vi "createBoolean.vi"(8 "error in (no error)":errorcluster, 10 "bool":bool, 11 "IBoolean in":refnum<class "IBoolean.lvclass">) -> (0 "error out":errorcluster, 3 "IBoolean out":refnum<class "IBoolean.lvclass">)   [LabVIEW 2022 SP3, in "openDAQ.lvlib" / "daqCoreTypes.lvlib" / "IBoolean.lvclass"]
uses:
  <instrlib>/openDAQ/Public/Classes/daqCoreTypes/IBoolean/IBoolean.lvclass
  C:/Program Files (x86)/National Instruments/LabVIEW 2022/instr.lib/openDAQ/Public/Classes/IBaseObject/IBaseObject.lvclass
  <instrlib>/openDAQ/Public/Classes/IBaseObject/IBaseObject.lvclass/IBaseObject.ctl
  <instrlib>/openDAQ/Public/Classes/IBaseObject/Accessor/Read reference.vi
  <instrlib>/openDAQ/Public/Classes/IBaseObject/Accessor/Write reference.vi
  <instrlib>/openDAQ/Binaries/Windows/x86/copendaq32.dll
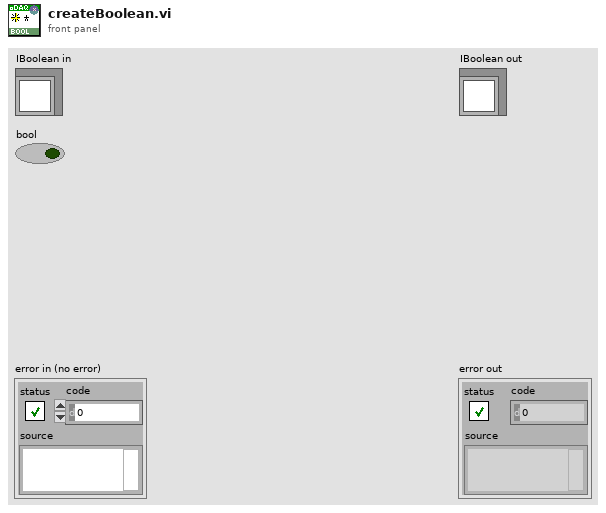
[diagram p1: front panel]
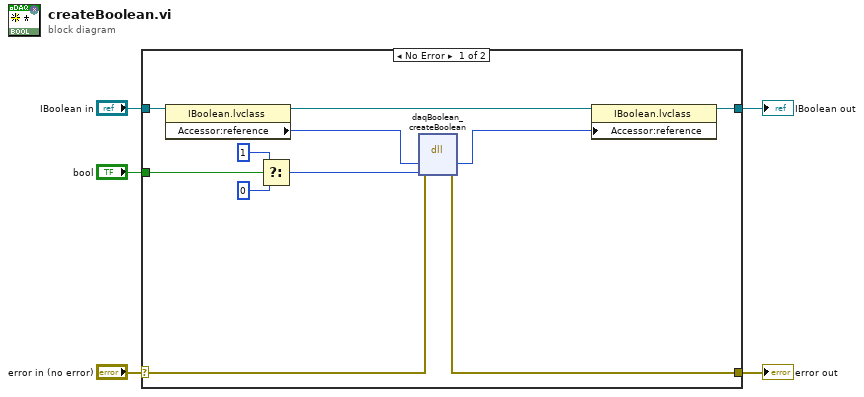
[diagram p0: block diagram]
diagram:
  n1 = case shown="No Error" "error in (no error)" {
    selector: "error in (no error)" -> [w16 w18]
    tunnel: [w15 w18] -> w4
    tunnel: [w13 w17] -> w2
    tunnel: "IBoolean in" -> [w14 w17]
    tunnel: "bool" -> [w9 _]
    frame No Error {
      n2 = property class="IBoolean.lvclass"(reference=w14) -> (reference out=w12:refnum<class "IBoolean.lvclass">, "Accessor:reference"=w11:i64)  [unwired: 1 in, 1 out]
      n3 = Select(t=i64 1 ("value"), s=w9, f=i64 0 ("value")) -> (s? t:f=w6:i64)
      n4 = dll-call lib="C:/Program Files (x86)/National Instruments/LabVIEW 2022/instr.lib/openDAQ/Binaries/Windows/x86/copendaq*.*" fn="daqBoolean_createBoolean"(error in=w16, "obj"=w11, "value"=w6) -> (error out=w15:errorcluster, "obj"=w10:i64)  [unwired: 4 in, 1 out]
      n5 = property class="IBoolean.lvclass"(reference=w12, "Accessor:reference"=w10) -> (reference out=w13:refnum<class "IBoolean.lvclass">)  [unwired: 1 in, 1 out]
    }
    frame Error {
    }
  }
  "error out" <- w4
  "IBoolean out" <- w2
